vi "Reporting_acqu.vi"(2 "output cluster":T1, 3 "address repoting":path) -> (1 "Reporting":string)   [LabVIEW 2015]
panel:
  out "error out":errorcluster
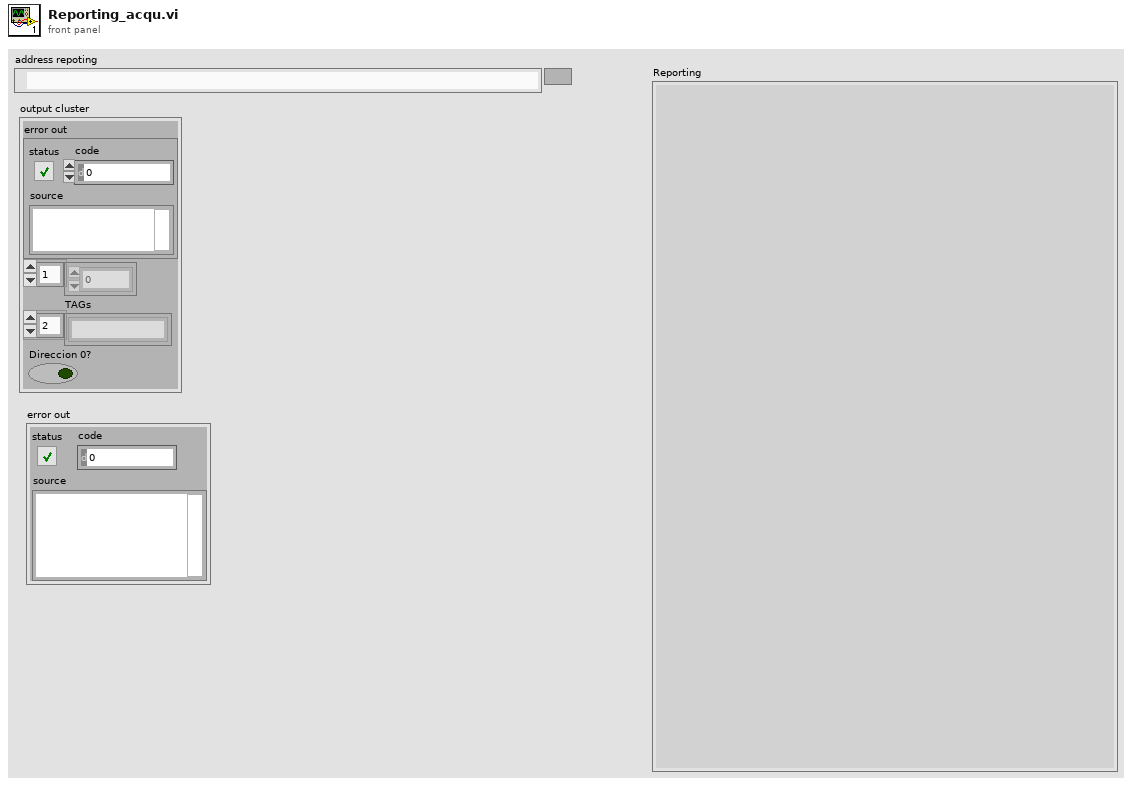
[diagram p1: front panel]
types:
  T1 = cluster{"error out":errorcluster, dbl[], "TAGs":string[], "Direccion 0?":bool}
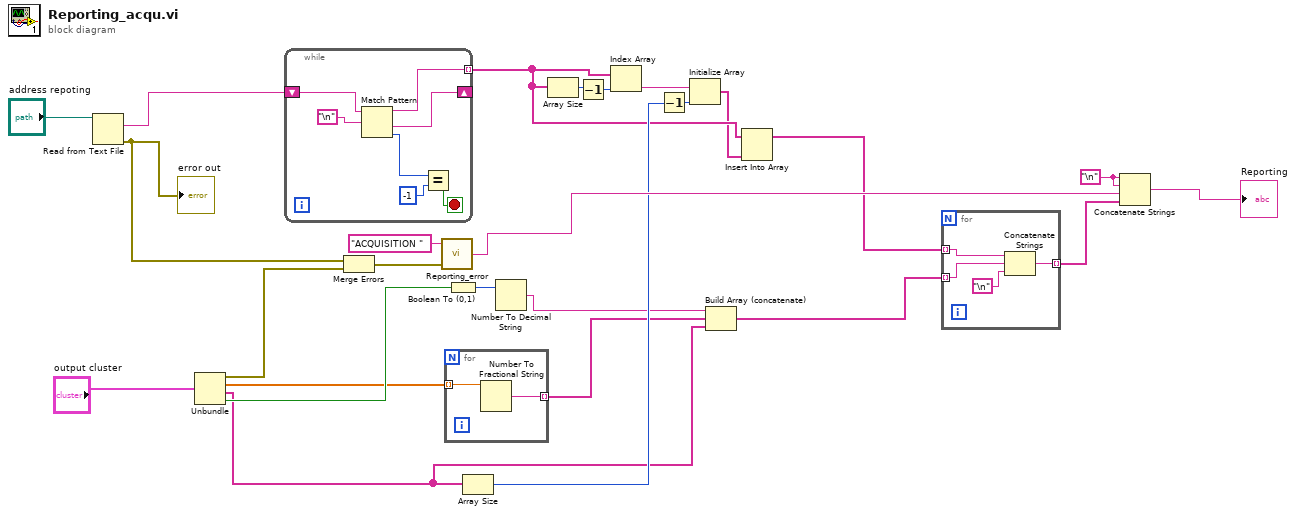
[diagram p0: block diagram]
diagram:
  w1 = "\n"
  n1 = Read from Text File(file (use dialog)="address repoting") -> (text=w26:string, error out=w21:errorcluster)  [unwired: 3 in, 2 out]
  "error out" <- w21
  n2 = Unbundle("output cluster") -> ("error out"=w20:errorcluster, w14:dbl[], "TAGs"=w3:string[], "Direccion 0?"=w16:bool)
  n3 = while {
    tunnel: [w30] -> w8 mode=indexing
    shift-right: [w27] -> _
    shift-left: w26 -> [w28]
    stop <- w33 stop-if-true
    n4 = Match Pattern(string=w28, regular expression="\n") -> (before substring=w30:string, after substring=w27:string, offset past match=w31:i32)  [unwired: 1 in, 1 out]
    n5 = Equal?(x=w31, y=-1) -> (x = y?=w33:bool)
  }
  n6 = Merge Errors(w21, w20) -> (w19:errorcluster)
  n7 = call "Reporting_error.vi"("error out 2"=w19, "Concept"="ACQUISITION ") -> ("Reporting"=w17:string)  [unwired: 1 in]
  n8 = for {
    tunnel: w14 -> [w35] mode=indexing
    tunnel: [w34] -> w4 mode=indexing
    n9 = Number To Fractional String(number=w35) -> (F-format string=w34:string)  [unwired: 3 in]
  }
  n10 = Boolean To (0,1)(Boolean=w16) -> (0, 1=w15:i16)
  n11 = Array Size(array=w3) -> (size(s)=w10:i32)
  n12 = Number To Decimal String(number=w15) -> (decimal integer string=w5:string)  [unwired: 1 in]
  n13 = Array Size(array=w8) -> (size(s)=w13:i32)
  n14 = Decrement(x=w13) -> (x-1=w12:i32)
  n15 = Index Array(array=w8, index=w12) -> (element=w11:string)
  n16 = Decrement(x=w10) -> (x-1=w9:i32)
  n17 = Initialize Array(w11, w9) -> (w7:string[])
  n18 = Build Array (concatenate)(w5, w4, w3) -> (w2:string[])
  n19 = Insert Into Array(array=w8, new element=w7) -> (w6:string[])  [unwired: 1 in]
  n20 = for {
    tunnel: w6 -> [w39] mode=indexing
    tunnel: w2 -> [w38] mode=indexing
    tunnel: [w36] -> w22 mode=indexing
    n21 = Concatenate Strings(w39, w38, "\n") -> (w36:string)
  }
  n22 = Concatenate Strings(w1, w1, w17, w22) -> (→"Reporting":string)
